vi "Const Lang Folder Path.vi"() -> (3 "Language Folder Path":path)   [LabVIEW 2018, in "Framework.lvlib" / "Framework.lvclass"]
uses:
  Framework/Framework/Framework.lvclass
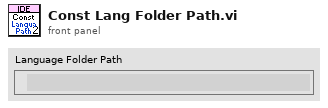
[diagram p1: front panel]
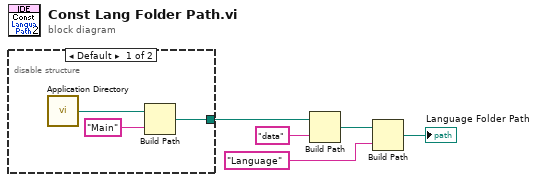
[diagram p0: block diagram]
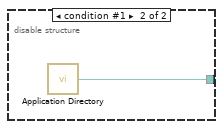
[diagram p2: hidden frame]
diagram:
  n1 = disable-structure shown="Default" {
    disable-tunnel: [w6 w9] -> w5
    frame condition #0 (active) {
      n2 = call <vilib>:"Application Directory.vi"() -> ("Application Directory"=w8:path)
      n3 = Build Path(base path=w8, name or relative path="Main") -> (appended path=w6:path)
    }
    frame condition #1 {
      n4 = call <vilib>:"Application Directory.vi"() -> ("Application Directory"=w9:path)
    }
  }
  n5 = Build Path(base path=w5, name or relative path="data") -> (appended path=w3:path)
  n6 = Build Path(base path=w3, name or relative path="Language") -> (appended path=→"Language Folder Path":path)
